vi "CalcAsterSize.vi"(1 "AsteroidData":T1={"Veloc"=0.0, "Direction"=0.0, "Size"=0, "displayRef"=refnum, "Max X"=0.0, "Max Y"=0.0, "Xpos"=0.0, "Ypos"=0.0, "ID"=0, "Config"={"SpaceShip"={"Angle"=30.0, "SideLenght"=2.0, "MaxLinearVeloc"=10.0, "MaxAngularVeloc"=10.0, "LinearAceleration"=1.0, "AngularAceleration"=1.0}, "Physics"={"LinearDragFactor"=1.0, "AngularDragFactor"=1.0}, "Asteroids"={"MaxSize"=6.0, "MaxDivisions"=3, "MaxVeloc"=8.0, "MinVeloc"=1.0, "Fill"=FALSE}, "Environment"={"MaxAsteroids"=10, "TimeIncrement"=0.1, "AsterProbCreation"=0.1, "LogEnabled"=FALSE}, "Shots"={"MinTimeShots"=10.0, "ShotSize"=0.1, "ShotSpeed"=0.1}}}) -> (0 "AsteroidSize":dbl)   [LabVIEW 2017]
uses:
  Asteroid_data.ctl
  GameConfig/GameConfig_data.ctl
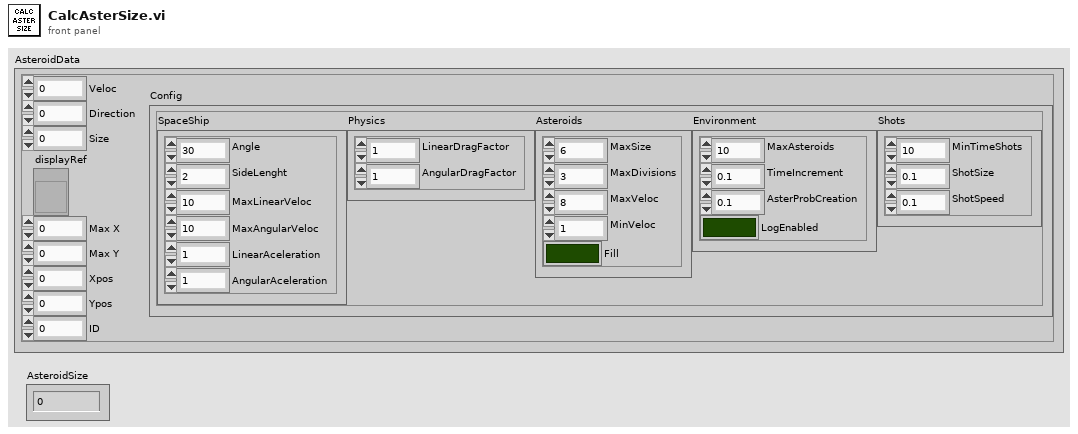
[diagram p1: front panel]
types:
  T1 = typedef "Asteroid_data.ctl" = cluster{"Veloc":dbl, "Direction":dbl, "Size":i32, "displayRef":refnum<vi>, "Max X":dbl, "Max Y":dbl, "Xpos":dbl, "Ypos":dbl, "ID":i32, "Config":T2}
  T2 = typedef "GameConfig_data.ctl" = cluster{"SpaceShip":cluster{"Angle":dbl, "SideLenght":dbl, "MaxLinearVeloc":dbl, "MaxAngularVeloc":dbl, "LinearAceleration":dbl, "AngularAceleration":dbl}, "Physics":cluster{"LinearDragFactor":dbl, "AngularDragFactor":dbl}, "Asteroids":cluster{"MaxSize":dbl, "MaxDivisions":i32, "MaxVeloc":dbl, "MinVeloc":dbl, "Fill":bool}, "Environment":cluster{"MaxAsteroids":i32, "TimeIncrement":dbl, "AsterProbCreation":dbl, "LogEnabled":bool}, "Shots":cluster{"MinTimeShots":dbl, "ShotSize":dbl, "ShotSpeed":dbl}}
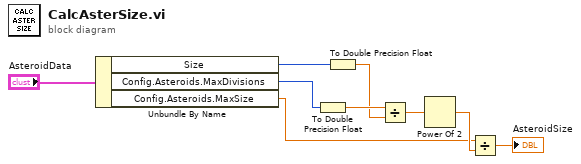
[diagram p0: block diagram]
diagram:
  n1 = Unbundle By Name("AsteroidData") -> ("Size"=w8:i32, "Config.Asteroids.MaxDivisions"=w2:i32, "Config.Asteroids.MaxSize"=w1:dbl)
  n2 = To Double Precision Float(number=w2) -> (double precision float=w7:dbl)
  n3 = To Double Precision Float(number=w8) -> (double precision float=w6:dbl)
  n4 = Divide(x=w7, y=w6) -> (x/y=w5:dbl)
  n5 = Power Of 2(x=w5) -> (2^x=w4:dbl)
  n6 = Divide(x=w1, y=w4) -> (x/y=→"AsteroidSize":dbl)
